vi "Write.vi"(6 "Append Index":i32, 8 "error in (no error)":errorcluster, 9 "Notes":string, 10 "Data (Dictionary)":T1[](array[typedef]), 11 "Data.ITX in":refnum<class "Data.ITX.lvclass">) -> (0 "error out":errorcluster, 3 "Data.ITX out":refnum<class "Data.ITX.lvclass">, 5 "Path out":path)   [LabVIEW 2020, in "Data.ITX.lvclass"]
uses:
  Data.ITX.lvclass
  C:/user/patrick/git/LV-to-ITX/src/Data/Data.lvclass
  Data/Typedefs/Dictionary--cluster.ctl
  Data/Data.lvclass/Data.ctl
  Data.ITX.lvclass/Data.ITX.ctl
  Data/Data.lvclass
  ITX Commands/ITX Commands.lvclass
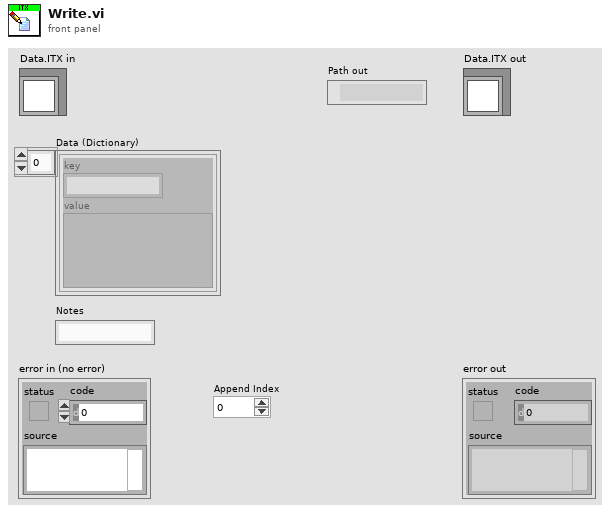
[diagram p1: front panel]
types:
  T1 = typedef "Data.lvclass/Dictionary--cluster.ctl" = cluster{"key":string, "value":variant}
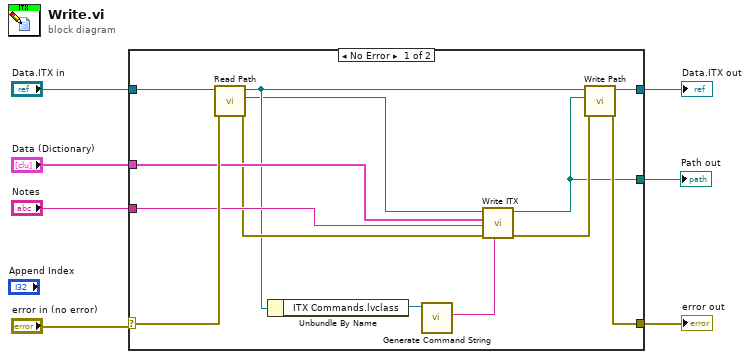
[diagram p0: block diagram]
diagram:
  n1 = case shown="No Error" "error in (no error)" {
    selector: "error in (no error)" -> [w19 w22]
    tunnel: [w17 w22] -> w4
    tunnel: "Data.ITX in" -> [w20 w21]
    tunnel: [w18 w21] -> w5
    tunnel: "Data (Dictionary)" -> [w15 _]
    tunnel: "Notes" -> [w14 _]
    tunnel: [w12 _] -> w1
    frame No Error {
      n2 = call "Read Path.vi"("error in (no error)"=w19, "Data Save"=w20) -> ("error out"=w13:errorcluster, "Path"=w8:path, "Data Save out"=w11:refnum<class "Data.ITX.lvclass">)  [unwired: 7 in]
      n3 = Unbundle By Name(w11) -> ("ITX Commands.lvclass"=w10:refnum<class "ITX Commands.lvclass">)
      n4 = call "Generate Command String.vi"("ITX Commands in"=w10) -> ("ITX Commands"=w9:string)  [unwired: 7 in, 2 out]
      n5 = call "Write ITX.vi"("Commands"=w9, "error in"=w13, "Notes"=w14, "Data (Dictionary)"=w15, "filename"=w8) -> ("error out"=w16:errorcluster, "file"=w12:path)  [unwired: 5 in]
      n6 = call "Write Path.vi"("error in (no error)"=w16, "Path"=w12, "Data Save"=w11) -> ("error out"=w17:errorcluster, "Data Save out"=w18:refnum<class "Data.ITX.lvclass">)  [unwired: 7 in]
    }
    frame Error {
    }
  }
  "error out" <- w4
  "Data.ITX out" <- w5
  "Path out" <- w1
